vi "SeqMgr.Variables, Populate Variable Value.vi"(8 "error in":errorcluster, 10 "String":string, 11 "Variables":variant) -> (0 "error out":errorcluster, 2 "String Out":string, 3 "Variables Out":variant)   [LabVIEW 2024, in "EQMF.lvlib" / "SeqMgr.lvlib"]
uses:
  SeqMgr.lvlib
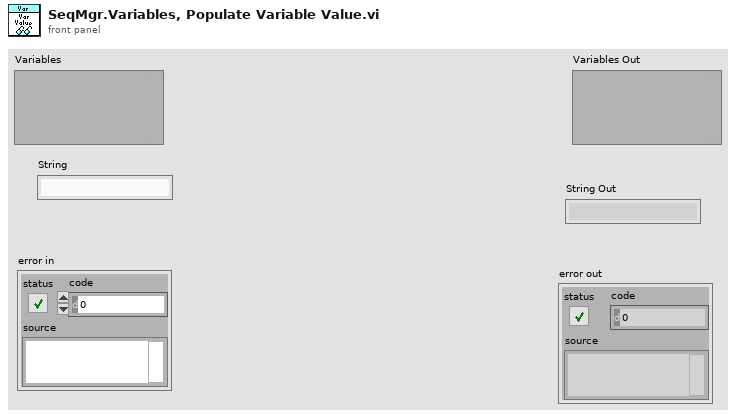
[diagram p1: front panel]
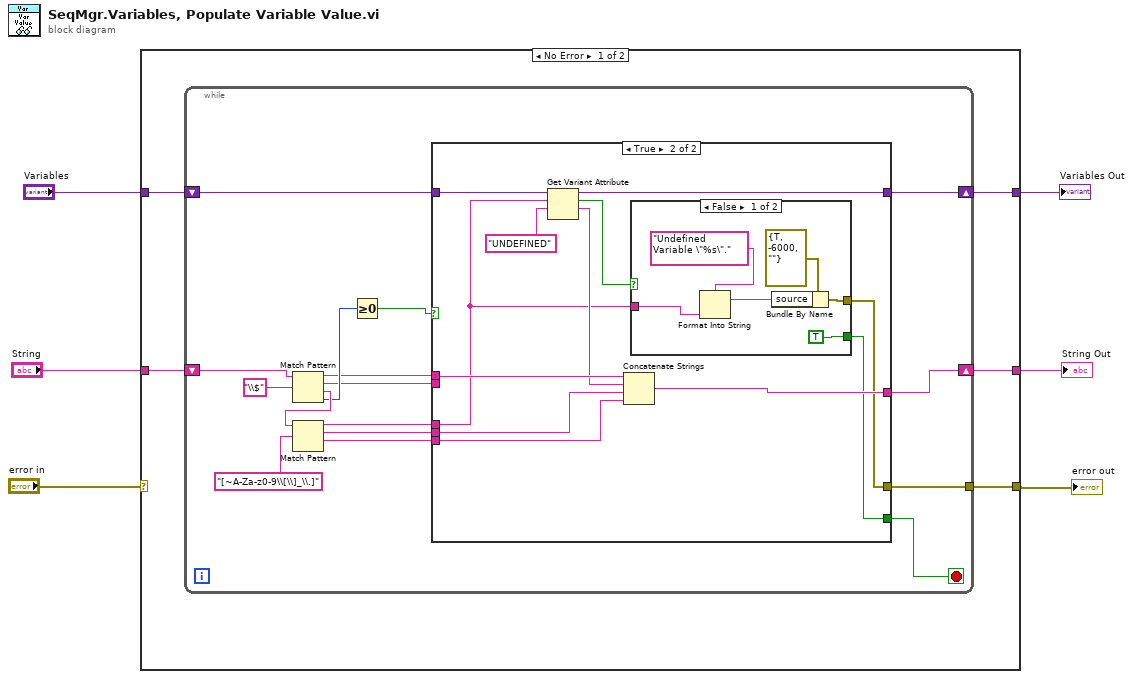
[diagram p0: block diagram]
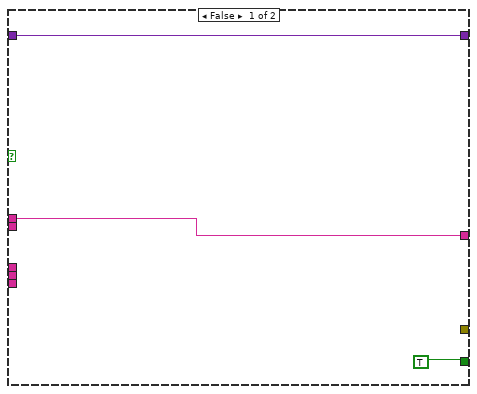
[diagram p2: hidden frame]
diagram:
  n1 = case shown="No Error" "error in" {
    selector: "error in" -> [_ w49]
    tunnel: "Variables" -> [w11 w51]
    tunnel: [w10 w51] -> w6
    tunnel: "String" -> [w9 w50]
    tunnel: [w8 w50] -> w4
    tunnel: [w7 w49] -> w2
    frame No Error {
      n2 = while {
        shift-right: [w26] -> w10
        shift-left: w11 -> [w27]
        shift-right: [w15] -> w8
        shift-left: w9 -> [w21]
        tunnel: [w13] -> w7
        stop <- w14 stop-if-true
        n3 = Match Pattern(string=w21, regular expression="\\$") -> (before substring=w19:string, match substring=w18:string, after substring=w23:string, offset past match=w22:i32)  [unwired: 1 in]
        n4 = Match Pattern(string=w23, regular expression="[~A-Za-z0-9\\[\\]_\\.]") -> (before substring=w20:string, match substring=w17:string, after substring=w16:string)  [unwired: 1 in, 1 out]
        n5 = Greater Or Equal To 0?(x=w22) -> (x >= 0?=w12:bool)
        n6 = case shown="True" w12 {
          tunnel: w27 -> [w28 w42]
          tunnel: [w28 w41] -> w26
          tunnel: w20 -> [_ w32]
          tunnel: w19 -> [w29 w39]
          tunnel: w18 -> [_ _]
          tunnel: w17 -> [_ w31]
          tunnel: w16 -> [_ w37]
          tunnel: [w29 w36] -> w15
          tunnel: [TRUE w34] -> w14
          tunnel: [_ w33] -> w13
          frame False {
          }
          frame True {
            n7 = Get Variant Attribute(Variant=w42, name=w32, default value (empty Variant)="UNDEFINED") -> (duplicate Variant=w41:variant, found=w35:bool, value=w38:string)  [unwired: 1 in, 1 out]
            n8 = Concatenate Strings(w39, w38, w31, w37) -> (w36:string)
            n9 = case shown="False" w35 {
              tunnel: [TRUE _] -> w34
              tunnel: [w46 _] -> w33
              tunnel: w32 -> [w44 _]
              frame False {
                n10 = Format Into String(format string="Undefined Variable \"%s\"." ("source"), w44) -> (resulting string=w43:string)  [unwired: 2 in, 1 out]
                n11 = Bundle By Name(cluster=errorcluster {"status"=TRUE, "code"=-6000, "source"=""} ("error constant"), "source"=w43) -> (w46:errorcluster)
              }
              frame True {
              }
            }
          }
        }
      }
    }
    frame Error {
    }
  }
  "Variables Out" <- w6
  "String Out" <- w4
  "error out" <- w2
